vi "Main.vi"() -> ()   [LabVIEW 2013]
uses:
  C:/Users/Andrew/Documents/Apatite to Zircon Code/LabVIEW and VB/LabVIEW and VB/LabVIEW and VB/bin/Release/LabVIEW and VB.dll
  LabVIEW and VB/LabVIEW and VB/bin/Release/LabVIEW and VB.dll
panel:
  out "_number2":dbl
  out "buildArray":i32[](array[numeric])
  out "addArrayElements":i32
  out "specialStringLength":i32
  in  "number2":dbl
  in  "number1":i32
  out "multiply":dbl
  out "add":i32
  out "error out":errorcluster
  in  "error in (no error)":errorcluster
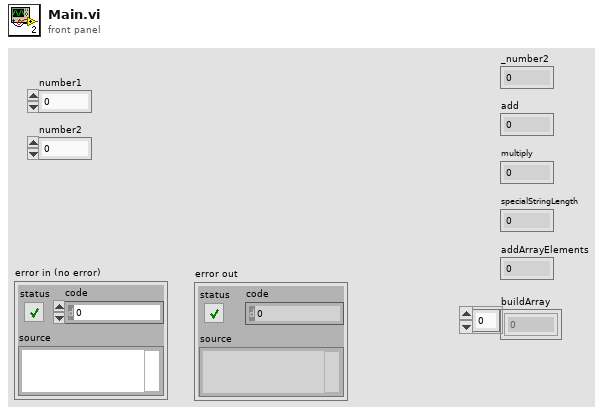
[diagram p1: front panel]
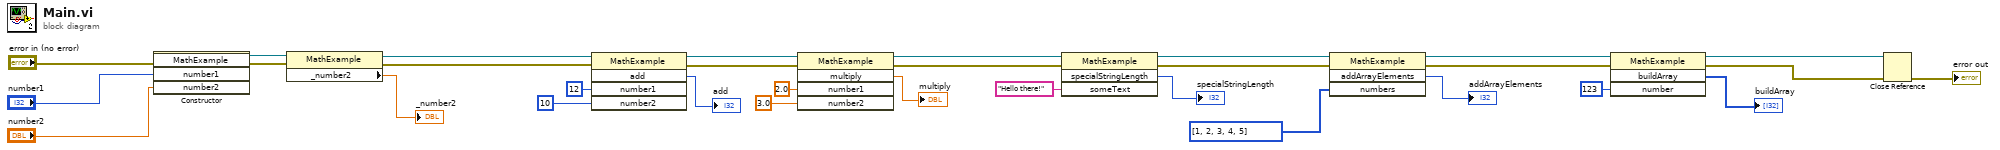
[diagram p0: block diagram]
diagram:
  n1 = constructor class="MathExample"(error in="error in (no error)", "number1"="number1", "number2"="number2") -> (reference out=w30:refnum<k24>, error out=w29:errorcluster)  [unwired: 2 in, 3 out]
  n2 = property class="MathExample"(reference=w30, error in=w29) -> (reference out=w28:refnum<k24>, error out=w27:errorcluster, "_number2"=→"_number2":dbl)
  n3 = invoke class="MathExample" method="add"(reference=w28, error in=w27, "number1"=12, "number2"=10) -> (reference out=w23:refnum<k24>, error out=w22:errorcluster, "add"=→"add":i32)  [unwired: 1 in, 2 out]
  n4 = invoke class="MathExample" method="multiply"(reference=w23, error in=w22, "number1"=2.0, "number2"=3.0) -> (reference out=w16:refnum<k24>, error out=w15:errorcluster, "multiply"=→"multiply":dbl)  [unwired: 1 in, 2 out]
  n5 = invoke class="MathExample" method="specialStringLength"(reference=w16, error in=w15, "someText"="Hello there!") -> (reference out=w12:refnum<k24>, error out=w11:errorcluster, "specialStringLength"=→"specialStringLength":i32)  [unwired: 1 in, 1 out]
  n6 = invoke class="MathExample" method="addArrayElements"(reference=w12, error in=w11, "numbers"=i32[] [1, 2, 3, 4, 5]) -> (reference out=w8:refnum<k24>, error out=w7:errorcluster, "addArrayElements"=→"addArrayElements":i32)  [unwired: 1 in, 1 out]
  n7 = invoke class="MathExample" method="buildArray"(reference=w8, error in=w7, "number"=123) -> (reference out=w4:refnum<k24>, error out=w3:errorcluster, "buildArray"=→"buildArray":i32[])  [unwired: 1 in, 1 out]
  n8 = Close Reference(reference=w4, error in (no error)=w3) -> (error out=→"error out":errorcluster)
